vi "DC microCurrent Configuration.vi"(8 "error in (no error)":errorcluster, 10 "uCurrent Range":T1, 11 "VISA resource name":refnum<visa-resource-name>) -> (0 "error out":errorcluster, 3 "VISA resource name out":refnum<visa-resource-name>)   [LabVIEW 2015, in "Keysight U1252.lvlib"]
uses:
  <instrlib>/Keysight U1252/Keysight U1252.lvlib
  <instrlib>/Keysight U1252/Controls/Micro Current Range.ctl
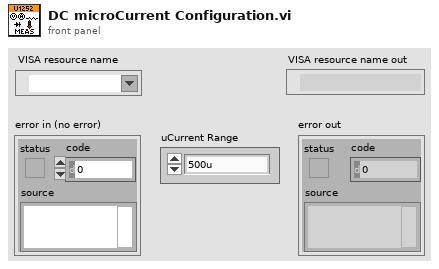
[diagram p1: front panel]
types:
  T1 = typedef "Keysight U1252.lvlib/Micro Current Range.ctl" = enum16{"500u", "5000u", "Auto"}
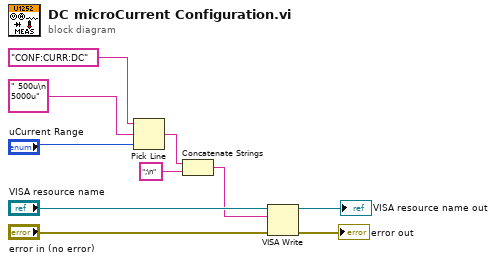
[diagram p0: block diagram]
diagram:
  n1 = Pick Line(string ("")="CONF:CURR:DC", multi-line string=" 500u\n 5000u", line index="uCurrent Range") -> (output string=w4:string)
  n2 = Concatenate Strings(w4, ";\n" ("string")) -> (w2:string)
  n3 = VISA Write(VISA resource name="VISA resource name", write buffer=w2, error in (no error)="error in (no error)") -> (VISA resource name out=→"VISA resource name out":refnum<visa-resource-name>, error out=→"error out":errorcluster)  [unwired: 1 out]
